vi "ViHandler.AsynchronusCall.vi"(4 "WaitUntilRegistered?":bool, 5 "CheckForExisting?":bool=TRUE, 7 "Modes":T2, 8 "Error In":errorcluster, 10 "ViQueueName(onlyForClones)":string, 11 "ViReference":refnum<vi>) -> (0 "error out":errorcluster, 1 "ViInfo(OnlyIfFound=true)":T1, 2 "ViFound?":bool, 3 "ViReference":refnum<vi>)   [LabVIEW 2016, in "ViHandler.lvclass"]
uses:
  ViHandler.lvclass
  ViHandler.RunModes.ctl
  ViHandler.ViInfo.ctl
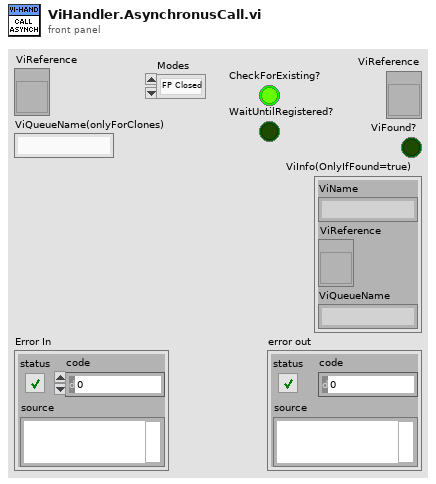
[diagram p1: front panel]
types:
  T1 = typedef "ViHandler.lvclass/ViHandler.ViInfo.ctl" = cluster{"ViName":string, "ViReference":refnum<vi>, "ViQueueName":string}
  T2 = typedef "ViHandler.lvclass/ViHandler.RunModes.ctl" = enum16{"FP Closed", "FP Open", "FP Open, Centered"}
  T3 = enum32{"Invalid", "Standard", "Closed", "Hidden", "Minimized", "Maximized"}
  T4 = enum32{"Bad", "Idle", "Run top level", "Running"}
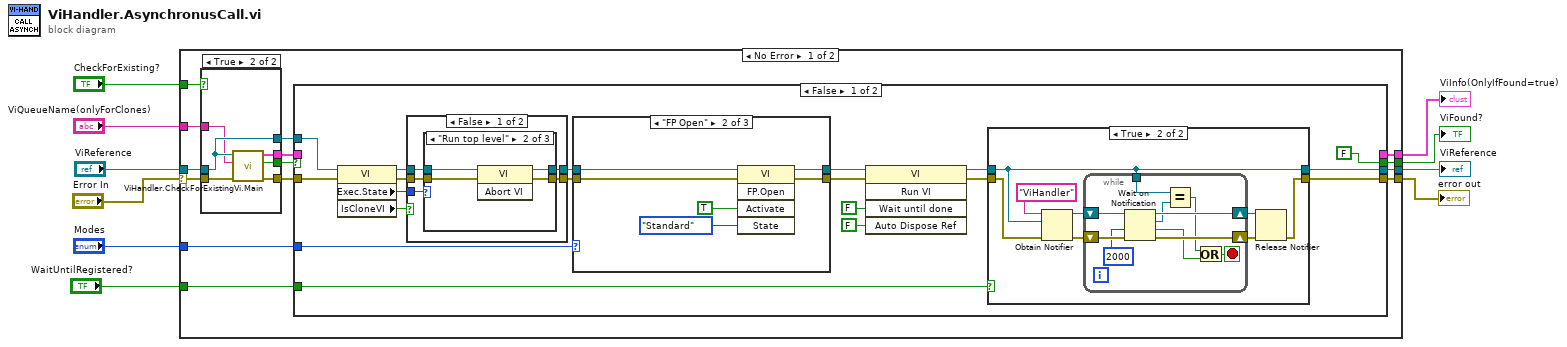
[diagram p0: block diagram]
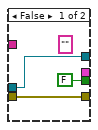
[diagram p2: hidden frame]
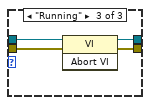
[diagram p5: hidden frame]
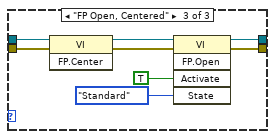
[diagram p8: hidden frame]
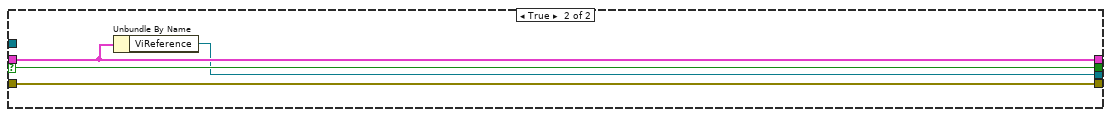
[diagram p9: hidden frame]
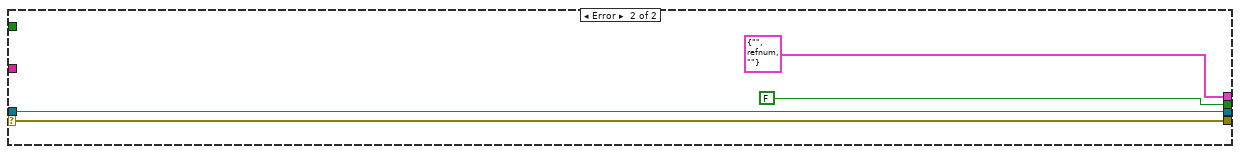
[diagram p10: hidden frame]
diagram:
  n1 = case shown="No Error" "Error In" {
    selector: "Error In" -> [w20 w113]
    tunnel: "ViReference" -> [w21 w112]
    tunnel: [w22 w112] -> w6
    tunnel: [w23 w113] -> w8
    tunnel: "Modes" -> [w24 _]
    tunnel: [w16 T1 {"ViName"="", "ViReference"=refnum, "ViQueueName"=""} ("ViInfo")] -> w4
    tunnel: [w15 FALSE] -> w5
    tunnel: "ViQueueName(onlyForClones)" -> [w14 _]
    tunnel: "CheckForExisting?" -> [w13 _]
    tunnel: "WaitUntilRegistered?" -> [w11 _]
    frame No Error {
      n2 = case shown="True" w13 {
        tunnel: w21 -> [w27 w29]
        tunnel: w20 -> [w25 w33]
        tunnel: [w25 w32] -> w19
        tunnel: [FALSE ("Found?") w31] -> w18
        tunnel: [_ w30] -> w17
        tunnel: w14 -> [_ w28]
        tunnel: [w27 w29] -> w12
        frame False {
          (unwired) "" ("ViQueueName(onlyForClones)")
        }
        frame True {
          n3 = call "ViHandler.CheckForExistingVi.Main.vi"("ErrorIn"=w33, "ViQueueName"=w28, "ViReference"=w29) -> ("ErrorOut"=w32:errorcluster, "Found?"=w31:bool, "ViInfo"=w30:T1)  [unwired: 6 in]
        }
      }
      n4 = case shown="False" w18 {
        selector: w18 -> [_ w108]
        tunnel: w24 -> [w52 _]
        tunnel: [w35 w109] -> w23
        tunnel: [w34 w106] -> w22
        tunnel: w12 -> [w42 _]
        tunnel: w19 -> [w41 w109]
        tunnel: w17 -> [_ w107]
        tunnel: [_ w107] -> w16
        tunnel: [FALSE w108] -> w15
        tunnel: w11 -> [w38 _]
        frame False {
          n5 = property class="VI"(reference=w42, error in=w41) -> (reference out=w45:refnum<vi>, error out=w44:errorcluster, "Exec.State"=w43:T4, "IsCloneVI"=w39:bool)
          n6 = case shown="False" w39 {
            tunnel: [w77 w89] -> w47
            tunnel: [w76 w88] -> w46
            tunnel: w45 -> [w75 w89]
            tunnel: w44 -> [w74 w88]
            tunnel: w43 -> [w73 _]
            frame False {
              n7 = case shown="\"Run top level\"" w73 {
                tunnel: [w79 w83 w87] -> w77
                tunnel: [w78 w82 w86] -> w76
                tunnel: w75 -> [w79 w81 w85]
                tunnel: w74 -> [w78 w80 w84]
                frame "Bad", Default {
                }
                frame "Run top level" {
                  n8 = invoke class="VI" method="Abort VI"(reference=w81, error in=w80) -> (reference out=w83:refnum<vi>, error out=w82:errorcluster)  [unwired: 1 in, 1 out]
                }
                frame "Running" {
                  n9 = invoke class="VI" method="Abort VI"(reference=w85, error in=w84) -> (reference out=w87:refnum<vi>, error out=w86:errorcluster)  [unwired: 1 in, 1 out]
                }
              }
            }
            frame True {
            }
          }
          n10 = case shown="\"FP Open\"" w52 {
            tunnel: w47 -> [w90 w93 w104]
            tunnel: [w90 w95 w101] -> w51
            tunnel: w46 -> [w91 w92 w100]
            tunnel: [w91 w94 w98] -> w50
            frame "FP Closed", Default {
            }
            frame "FP Open" {
              n11 = invoke class="VI" method="FP.Open"(reference=w93, error in=w92, "Activate"=TRUE ("Activate?"), "State"=T3."Standard") -> (reference out=w95:refnum<vi>, error out=w94:errorcluster)  [unwired: 1 in, 3 out]
            }
            frame "FP Open, Centered" {
              n12 = invoke class="VI" method="FP.Center"(reference=w104, error in=w100) -> (reference out=w105:refnum<vi>, error out=w99:errorcluster)  [unwired: 1 in, 1 out]
              n13 = invoke class="VI" method="FP.Open"(reference=w105, error in=w99, "Activate"=TRUE ("Activate?"), "State"=T3."Standard") -> (reference out=w101:refnum<vi>, error out=w98:errorcluster)  [unwired: 1 in, 3 out]
            }
          }
          n14 = invoke class="VI" method="Run VI"(reference=w51, error in=w50, "Wait until done"=FALSE ("Wait Until Done"), "Auto Dispose Ref"=FALSE ("Auto Dispose Reference")) -> (reference out=w36:refnum<vi>, error out=w37:errorcluster)  [unwired: 1 in, 3 out]
          n15 = case shown="True" w38 {
            tunnel: w37 -> [w53 w57]
            tunnel: w36 -> [w54 w56]
            tunnel: [w53 w55] -> w35
            tunnel: [w54 w56] -> w34
            frame False {
            }
            frame True {
              n16 = Obtain Notifier(name (unnamed)="ViHandler", notification data type=w56, error in (no error)=w57) -> (notifier out=w60:refnum<notifier>, error out=w59:errorcluster)  [unwired: 1 in, 1 out]
              n17 = while {
                shift-right: [w72] -> w61
                shift-left: w60 -> [w71]
                shift-right: [w69] -> w58
                shift-left: w59 -> [w70]
                tunnel: w56 -> [w64]
                stop <- w67 stop-if-true
                n18 = Wait on Notification(notifier=w71, timeout in ms (-1)=2000, error in (no error)=w70) -> (notifier out=w72:refnum<notifier>, notification=w65:refnum<vi>, timed out?=w66:bool, error out=w69:errorcluster)  [unwired: 1 in]
                n19 = Equal?(x=w64, y=w65) -> (x = y?=w63:bool)
                n20 = Or(x=w63, y=w66) -> (x .or. y?=w67:bool)
              }
              n21 = Release Notifier(notifier=w61, error in (no error)=w58) -> (error out=w55:errorcluster)  [unwired: 1 in, 2 out]
            }
          }
        }
        frame True {
          n22 = Unbundle By Name(w107) -> ("ViReference"=w106:refnum<vi>)
        }
      }
    }
    frame Error {
    }
  }
  "error out" <- w8
  "ViReference" <- w6
  "ViFound?" <- w5
  "ViInfo(OnlyIfFound=true)" <- w4
